vi "FlatToRichnidaqmx_grpc_CreateTaskRequest.vi"(5 "OutputClusterType":T1, 11 "InputCluster":T3) -> (3 "OutputCluster":T1)   [LabVIEW 2021, in "NI DAQmx_server.lvlib"]
uses:
  NI DAQmx_server.lvlib
  nidaqmx_grpc_CreateTaskRequest_Flat.ctl
  nidevice_grpc_SessionInitializationBehavior.ctl
  nidaqmx_grpc_CreateTaskRequest.ctl
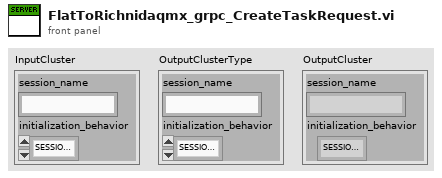
[diagram p1: front panel]
types:
  T1 = typedef "NI DAQmx_server.lvlib/nidaqmx_grpc_CreateTaskRequest.ctl" = cluster{"session_name":string, "initialization_behavior":T2}
  T2 = typedef "NI DAQmx_server.lvlib/nidevice_grpc_SessionInitializationBehavior.ctl" = enum32{"SESSION_INITIALIZATION_BEHAVIOR_UNSPECIFIED", "SESSION_INITIALIZATION_BEHAVIOR_INITIALIZE_NEW", "SESSION_INITIALIZATION_BEHAVIOR_ATTACH_TO_EXISTING"}
  T3 = typedef "NI DAQmx_server.lvlib/nidaqmx_grpc_CreateTaskRequest_Flat.ctl" = cluster{"session_name":string, "initialization_behavior":T2}
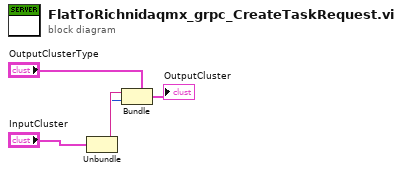
[diagram p0: block diagram]
diagram:
  n1 = Unbundle "Unbundle"("InputCluster") -> ("session_name"=w2:string, "initialization_behavior"=w1:T2)
  n2 = Bundle "Bundle"(cluster="OutputClusterType", "session_name"=w2, "initialization_behavior"=w1) -> (→"OutputCluster":T1)
